vi "Invert_Output_Lines.vi"(8 "Error In":errorcluster, 10 "Line Inversion Array":bool[](array[boolean]), 11 "VLIW Array In":T1(array[cluster])=[{"Output Bits"=0, "Data Field"=3, "OP Code"=2, "Delay Count"=4}, {"Output Bits"=0, "Data Field"=0, "OP Code"=3, "Delay Count"=4}, {"Output Bits"=0, "Data Field"=0, "OP Code"=0, "Delay Count"=2599999997}, {"Output Bits"=0, "Data Field"=2, "OP Code"=7, "Delay Count"=1073741821}, {"Output Bits"=0, "Data Field"=0, "OP Code"=0, "Delay Count"=705032701}] {"OP Code" format="%.0x"; "Output Bits" format="%.0x"}) -> (0 "Error Out":errorcluster, 3 "VLIW Array Out":T1(array[cluster])=[{"Output Bits"=0, "Data Field"=3, "OP Code"=2, "Delay Count"=4}, {"Output Bits"=0, "Data Field"=0, "OP Code"=3, "Delay Count"=4}, {"Output Bits"=0, "Data Field"=0, "OP Code"=0, "Delay Count"=2599999997}, {"Output Bits"=0, "Data Field"=2, "OP Code"=7, "Delay Count"=1073741821}, {"Output Bits"=0, "Data Field"=0, "OP Code"=0, "Delay Count"=705032701}] {"OP Code" format="%.0x"; "Output Bits" format="%.0x"})   [LabVIEW 2013, in "Pulseblaster.lvclass"]
uses:
  Pulseblaster.lvclass
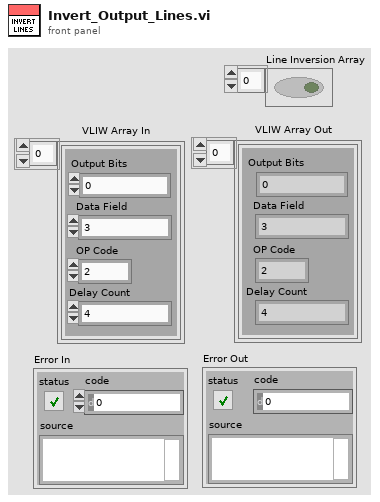
[diagram p1: front panel]
types:
  T1 = cluster{"Output Bits":u32, "Data Field":u32, "OP Code":u8, "Delay Count":u64}[]
  T2 = cluster{"Output Bits":u32, "Data Field":u32, "OP Code":u8, "Delay Count":u64}
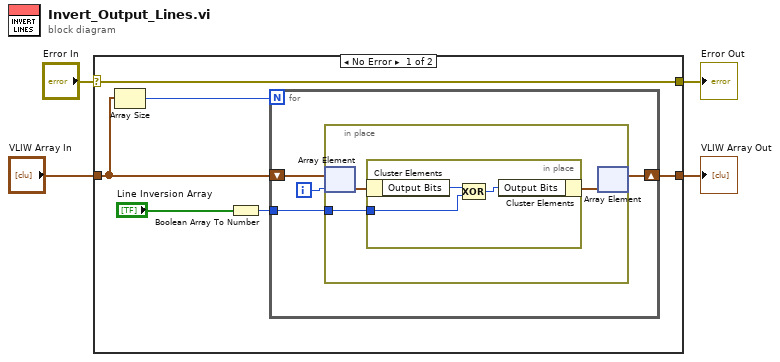
[diagram p0: block diagram]
diagram:
  n1 = case shown="No Error" "Error In" {
    selector: "Error In" -> [w5 w21]
    tunnel: [w7 w22] -> w2
    tunnel: "VLIW Array In" -> [w6 w22]
    tunnel: [w5 w21] -> w4
    frame No Error {
      n2 = Array Size(array=w6) -> (size(s)=w10:i32)
      n3 = Boolean Array To Number(Boolean array="Line Inversion Array") -> (number=w9:u32)
      n4 = for {
        N: w10 -> [_]
        tunnel: w9 -> [w12]
        shift-right: [w11] -> w7
        shift-left: w6 -> [w14]
        i -> [w13]
        n5 = in-place {
          in-place-border: w12 -> [w15]
          n6 = in-place-array #1(w14, w13) -> (w16:T2)
          n7 = in-place {
            in-place-border: w15 -> [w18]
            n8 = in-place-cluster #2(w16) -> ("Output Bits"=w20:u32)
            n9 = Compound Arithmetic op=XOR(w20, w18) -> (w19:u32)
            n10 = in-place-cluster #2("Output Bits"=w19) -> (w17:T2)
          }
          n11 = in-place-array #1(w17) -> (w11:T1)  [unwired: 1 out]
        }
      }
    }
    frame Error {
    }
  }
  "Error Out" <- w4
  "VLIW Array Out" <- w2
